vi "alarmBeep.vi"(11 "Alarm?":bool) -> ()   [LabVIEW 2017]
panel:
  in  "SpeechLib.ISpeechVoice":refnum<k7>
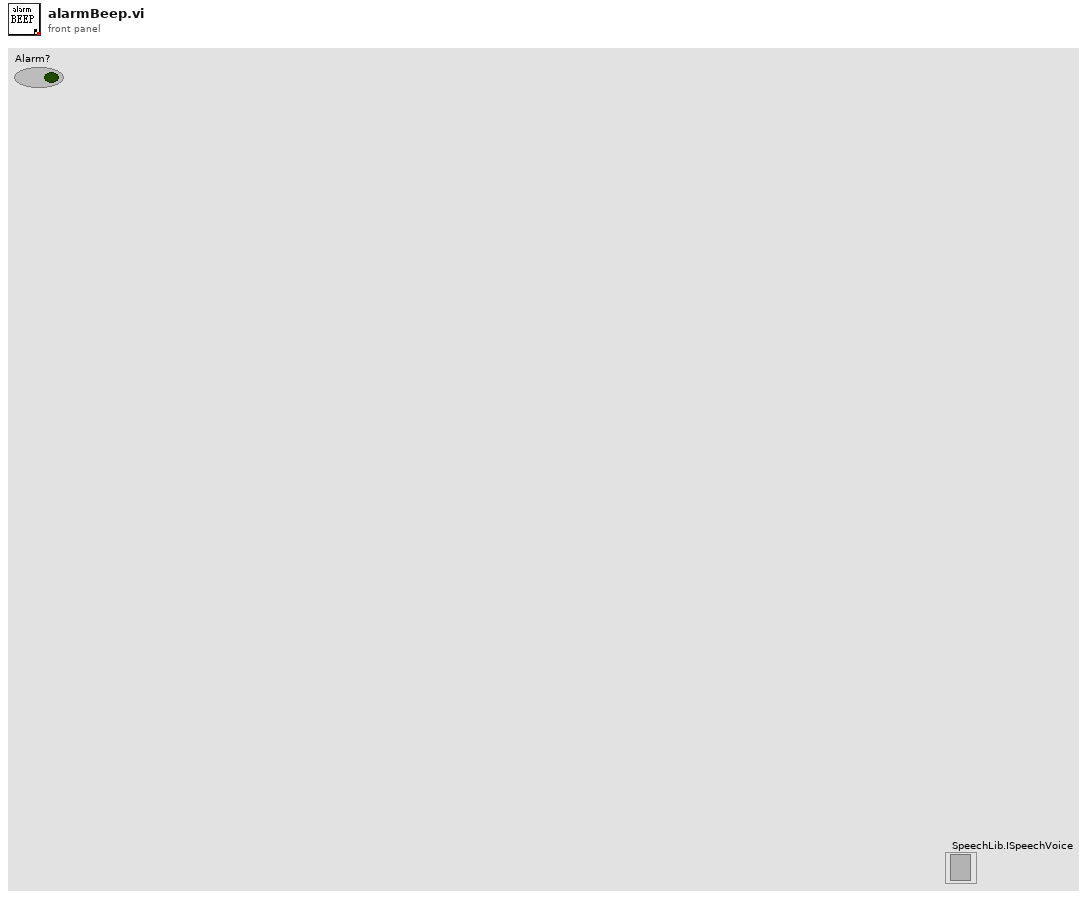
[diagram p1: front panel]
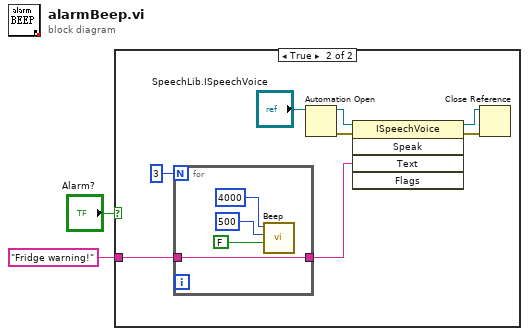
[diagram p0: block diagram]
diagram:
  n1 = case shown="True" "Alarm?" {
    tunnel: "Fridge warning!" ("Error msg") -> [_ w3]
    frame False {
    }
    frame True {
      n2 = for {
        N: 3 -> [_]
        tunnel: [w11] -> w4
        tunnel: w3 -> [w11]
        n3 = call <vilib>:"Beep.vi"("use system alert? (T)"=FALSE, "duration (msec)"=u32 500, "frequency (Hz)"=u32 4000) -> ()  [unwired: 9 out]
      }
      n4 = Automation Open(Automation Refnum="SpeechLib.ISpeechVoice") -> (Automation Refnum=w5:refnum<k7>, error out=w6:errorcluster)  [unwired: 1 in, 2 out]
      n5 = invoke class="ISpeechVoice" method="Speak"(reference=w5, error in=w6, "Text"=w4) -> (reference out=w8:refnum<k7>, error out=w9:errorcluster)  [unwired: 2 in, 3 out]
      n6 = Close Reference(reference=w8, error in (no error)=w9) -> ()  [unwired: 1 out]
    }
  }
